vi "Copy.vi"(8 "error in (no error)":errorcluster, 10 "dst":path, 11 "src":path) -> (0 "error out":errorcluster)   [LabVIEW 2014, in "lvprj2html.lvlib"]
uses:
  lvprj2html.lvlib
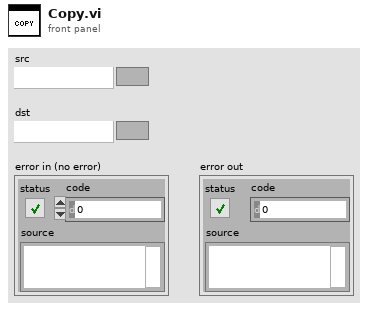
[diagram p1: front panel]
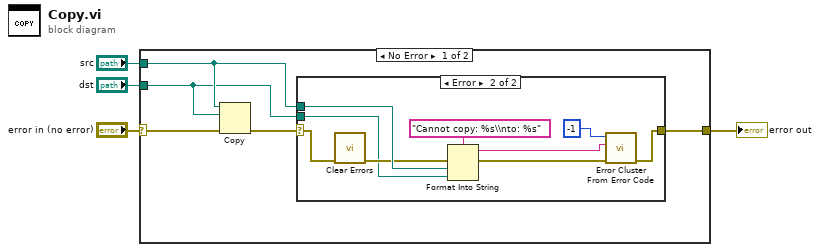
[diagram p0: block diagram]
diagram:
  n1 = case shown="No Error" "error in (no error)" {
    selector: "error in (no error)" -> [w9 w20]
    tunnel: [w7 w20] -> w4
    tunnel: "dst" -> [w5 _]
    tunnel: "src" -> [w6 _]
    frame No Error {
      n2 = Copy(8:w9, 10:w5, 11:w6) -> (0:w8:errorcluster)  [unwired: 2 in, 2 out]
      n3 = case shown="Error" w8 {
        selector: w8 -> [w10 w13]
        tunnel: w6 -> [_ w16]
        tunnel: [w10 w19] -> w7
        tunnel: w5 -> [_ w11]
        frame No Error {
        }
        frame Error {
          n4 = call <vilib>:"Clear Errors.vi"("error in (no error)"=w13) -> ("error out"=w12:errorcluster)  [unwired: 5 in, 1 out]
          n5 = Format Into String(format string="Cannot copy: %s\\nto: %s", error in=w12, w16, w11) -> (resulting string=w15:string, error out=w14:errorcluster)  [unwired: 1 in]
          n6 = call <vilib>:"Error Cluster From Error Code.vi"("error in (no error)"=w14, "error message (\"\")"=w15, "error code (0)"=-1) -> ("error out"=w19:errorcluster)  [unwired: 6 in]
        }
      }
    }
    frame Error {
    }
  }
  "error out" <- w4
